vi "test Remote IO DIO Loop Back.vi"(8 "error in (no error)":errorcluster, 11 "TestCase in":refnum<class "Scan Engine EtherCAT System Tests.lvclass">) -> (0 "error out":errorcluster, 3 "TestCase out":refnum<class "Scan Engine EtherCAT System Tests.lvclass">)   [LabVIEW 2019, in "Scan Engine EtherCAT System Tests.lvclass"]
uses:
  Scan Engine EtherCAT System Tests.lvclass
  C:/Users/nitest/Desktop/Git 2019/niveristand-custom-device-testing-tools/VeriStandTestCase/VeriStandTestCase.lvclass
  <vilib>/addons/_JKI Toolkits/VI Tester/TestCase.llb/TestCase.lvclass
  niveristand-custom-device-testing-tools/VeriStandTestCase/VeriStandTestCase.lvclass
  C:/Program Files (x86)/National Instruments/LabVIEW 2019/vi.lib/addons/_JKI Toolkits/VI Tester/TestCase.llb/TestCase.lvclass
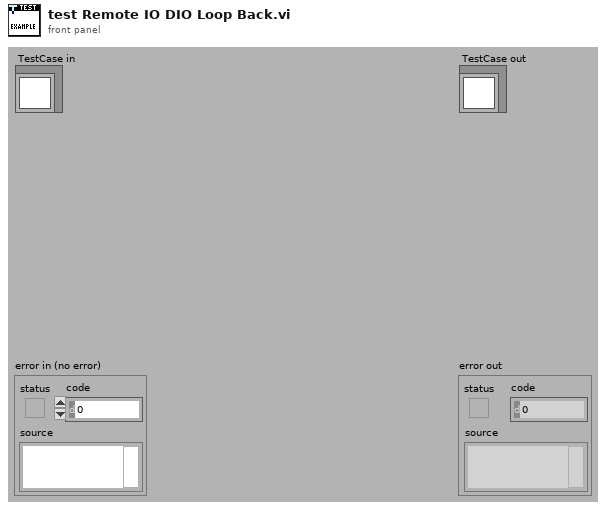
[diagram p1: front panel]
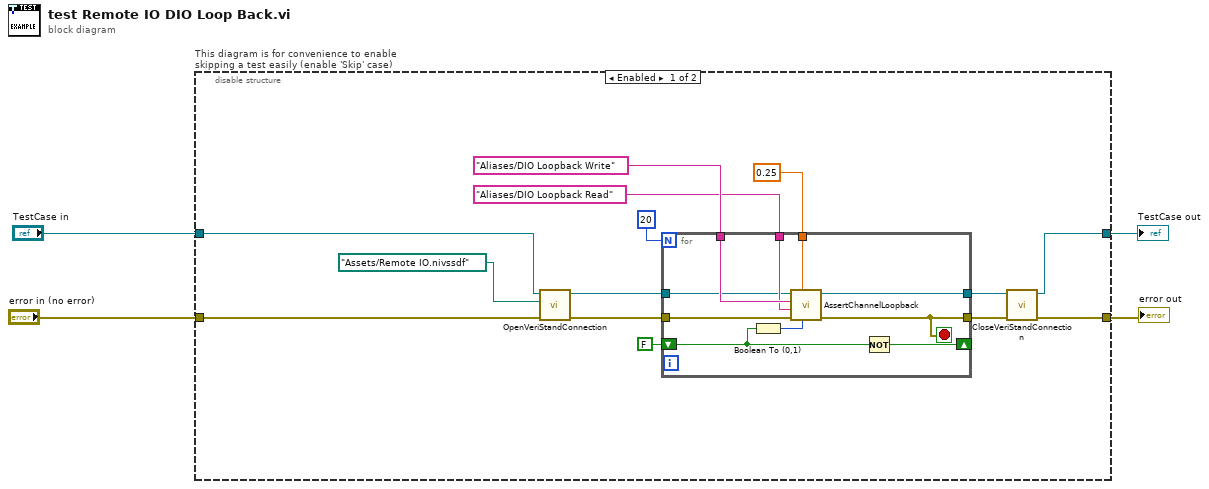
[diagram p0: block diagram]
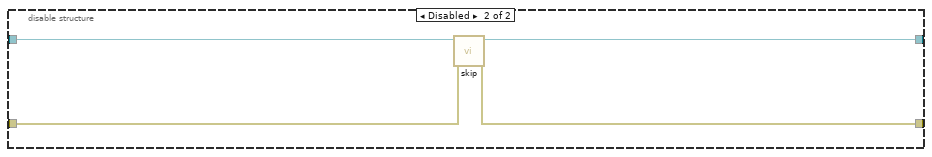
[diagram p2: hidden frame]
diagram:
  n1 = disable-structure "This diagram is for convenience to enable skipping a test easily (enable 'Skip' case)" shown="Enabled" {
    disable-tunnel: "TestCase in" -> [w7 w32]
    disable-tunnel: [w6 w30] -> w1
    disable-tunnel: [w9 w31] -> w3
    disable-tunnel: "error in (no error)" -> [w8 w29]
    frame Enabled {
      n2 = call-dynamic "OpenVeriStandConnection.vi"("error in (no error)"=w8, "System Definition File"=path "Assets/Remote IO.nivssdf", "VeriStand Test Case in"=w7) -> ("error out"=w13:errorcluster, "VeriStand Test Case out"=w12:refnum<class "Scan Engine EtherCAT System Tests.lvclass">)  [unwired: 6 in, 1 out]
      n3 = for {
        N: 20 -> [_]
        tunnel: "Aliases/DIO Loopback Write" ("Channel") -> [w25]
        tunnel: [w23] -> w11
        tunnel: "Aliases/DIO Loopback Read" ("Channel") -> [w24]
        shift-right: [w28] -> _
        shift-left: FALSE -> [w27]
        tunnel: w13 -> [w26]
        tunnel: [w20] -> w10
        tunnel: w12 -> [w21]
        tunnel: 0.25 ("Delay Time (s)") -> [w19]
        stop <- w23 stop-if-true
        n4 = Boolean To (0,1)(Boolean=w27) -> (0, 1=w22:i16)
        n5 = call "AssertChannelLoopback.vi"("Value"=w22, "Delay Time (s)"=w19, "error in (no error)"=w26, "Read Channel"=w24, "Write Channel"=w25, "VeriStand Test Case in"=w21) -> ("error out"=w23:errorcluster, "VeriStand Test Case out"=w20:refnum<class "Scan Engine EtherCAT System Tests.lvclass">)  [unwired: 4 in]
        n6 = Not(x=w27) -> (.not. x?=w28:bool)
      }
      n7 = call-dynamic "CloseVeriStandConnection.vi"("error in (no error)"=w11, "VeriStand Test Case in"=w10) -> ("error out"=w9:errorcluster, "VeriStand Test Case out"=w6:refnum<class "Scan Engine EtherCAT System Tests.lvclass">)  [unwired: 8 in]
    }
    frame Disabled {
      n8 = call <vilib>:"skip.vi"("error in (no error)"=w29, "TestCase in"=w32) -> ("error out"=w31:errorcluster, "TestCase out"=w30:refnum<class "Scan Engine EtherCAT System Tests.lvclass">)  [unwired: 8 in]
    }
  }
  "error out" <- w3
  "TestCase out" <- w1
